vi "Read configuration.vi"(8 "error in":errorcluster, 11 "tag select module editor node in":refnum<class "tag select module editor node.lvclass">) -> (0 "error out":errorcluster, 2 "configuration":refnum<class "NISE_CEF_serializable configuration.lvclass">, 3 "tag select module editor node out":refnum<class "tag select module editor node.lvclass">)   [LabVIEW 2015, in "tag select module editor node.lvclass"]
uses:
  tag select module editor node.lvclass
  <vilib>/NI/Configuration Framework/serializable configuration/NISE_CEF_serializable configuration.lvclass
  tag select module editor node.lvclass/tag select module editor node.ctl
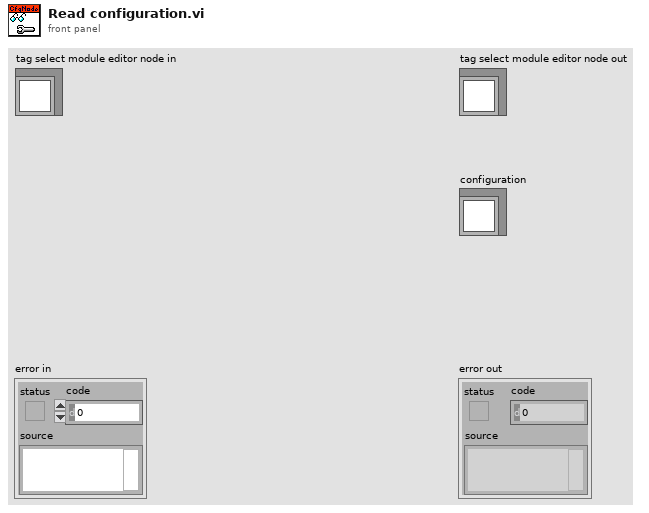
[diagram p1: front panel]
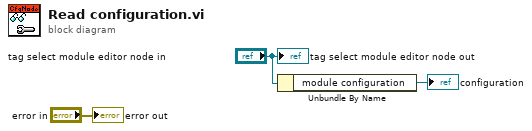
[diagram p0: block diagram]
diagram:
  n1 = Unbundle By Name("tag select module editor node in") -> ("module configuration"=→"configuration":refnum<class "tag select module configuration.lvclass">)
  "error out" <- "error in"
  "tag select module editor node out" <- "tag select module editor node in"
